vi "InitSignalDatabase.vi"(8 "error in":errorcluster, 11 "ConfigFile":path) -> (0 "error out":errorcluster, 3 "Trigger Data":T3)   [LabVIEW 2016]
uses:
  Ctrl_Signal.ctl
  Ctrl_Signal_Map.ctl
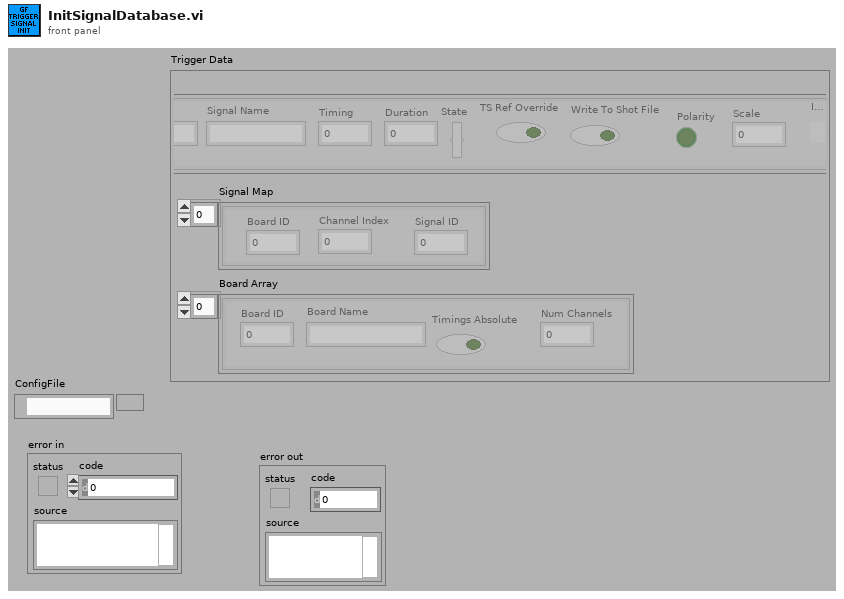
[diagram p1: front panel]
types:
  T1 = typedef "Ctrl_Signal.ctl" = cluster{"Signal Name":string, "Timing":dbl, "Duration":dbl, "State":bool, "TS Ref Override":bool, "Write To Shot File":bool, "Polarity":bool, "Signal ID":dbl, "Scale":dbl, "IsDelay":bool}
  T2 = typedef "Ctrl_Signal_Map.ctl" = cluster{"Channel Index":dbl, "Board ID":dbl, "Signal ID":dbl}
  T3 = cluster{"Signal Array":T1[], "Signal Map":T2[], "Board Array":cluster{"Board ID":dbl, "Board Name":string, "Timings Absolute":bool, "Num Channels":dbl}[]}
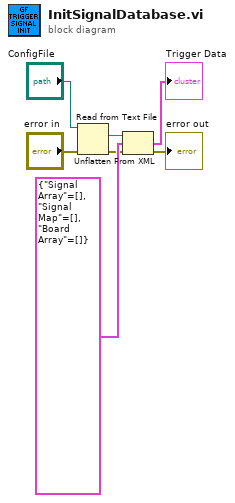
[diagram p0: block diagram]
diagram:
  n1 = Read from Text File(file (use dialog)="ConfigFile", error in="error in") -> (text=w5:string, error out=w3:errorcluster)  [unwired: 2 in, 2 out]
  n2 = Unflatten From XML(xml string=w5, type=T3 {"Signal Array"=[], "Signal Map"=[], "Board Array"=[]} ("Trigger Data"), error in (no error)=w3) -> (value=→"Trigger Data":T3, error out=→"error out":errorcluster)
